vi "Launch Devices to Load Dialog.vi"(8 "error in":errorcluster, 11 "Master Controller in":refnum<class "EMS User Interface.lvclass">) -> (0 "error out":errorcluster, 3 "Master Controller out":refnum<class "EMS User Interface.lvclass">)   [LabVIEW 2018, in "EMS User Interface Actor.lvlib" / "EMS User Interface.lvclass"]
uses:
  EMS User Interface.lvclass
  C:/Users/Administrator/Desktop/LabVIEW EMS/EMS Generic Actor/EMS Generic/EMS Generic.lvclass
  C:/Program Files (x86)/National Instruments/LabVIEW 2018/vi.lib/ActorFramework/Actor/Actor.lvclass
  Dialog Actors/Devices to Load Actor/Devices to Load/Devices to Load.lvclass
  EMS User Interface Messages/Write Device IDs Msg/Write Device IDs Msg.lvclass
  C:/Users/Administrator/Desktop/LabVIEW EMS/Dialog Actors/Devices to Load Actor/Devices to Load Messages/Return Devices to Load IDs Msg/Return Devices to Load IDs Msg.lvclass
  EMS Generic Actor/EMS Generic/EMS Generic.lvclass/EMS Generic.ctl
  EMS User Interface.lvclass/EMS User Interface.ctl
  Dialog Actors/Devices to Load Actor/Devices to Load Messages/Update Device List Msg/Update Device List Msg.lvclass/Update Device List Msg.ctl
  <vilib>/ActorFramework/Message Enqueuer/Message Enqueuer.lvclass/Message Enqueuer.ctl
  <vilib>/ActorFramework/Message Enqueuer/Enqueue.vi
  Dialog Actors/Devices to Load Actor/Devices to Load Messages/Update Device List Msg/Update Device List Msg.lvclass
  C:/Program Files (x86)/National Instruments/LabVIEW 2018/vi.lib/ActorFramework/Message/Message.lvclass
  Global Variables/Global Variables.vi
  <vilib>/ActorFramework/Message Priority Queue/Priority Enqueue.vi
  <vilib>/ActorFramework/Actor/Actor.lvclass
  EMS Generic Actor/EMS Generic/EMS Generic.lvclass
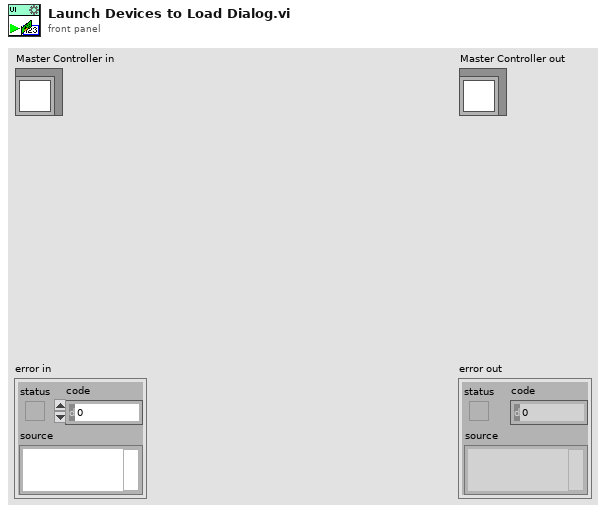
[diagram p1: front panel]
types:
  T1 = typedef "CSEISMIC DDS.lvlib/CSEISMIC DDS.lvclass/DeviceID.ctl" = string
  T2 = typedef "EMS Generic Actor.lvlib/EMS Generic.lvclass/Data Type DVRs.ctl" = cluster{"IED_Status":refnum<data-value>, "IED_Status_0":refnum<data-value>, "DER_Measurement":refnum<data-value>, "DER_Info":refnum<data-value>, "DER_Status":refnum<data-value>, "ES_Measurement":refnum<data-value>, "ES_Info":refnum<data-value>, "PV_Info":refnum<data-value>, "SmartRelay_Info":refnum<data-value>, "SmartRelay_Measurement":refnum<data-value>, "Meter_Info":refnum<data-value>, "Meter_Measurement":refnum<data-value>, "HVAC_Status":refnum<data-value>, "HVAC_Measurement":refnum<data-value>, "PriceData_RealTime":refnum<data-value>, "PriceData_Demand":refnum<data-value>, "PriceData_Energy":refnum<data-value>, "ForecastData_Long":refnum<data-value>, "ForecastData_Short":refnum<data-value>, "DER_Control":refnum<data-value>, "DER_SetPointF":refnum<data-value>, "DER_SetPointP":refnum<data-value>, "DER_SetPointQ":refnum<data-value>, "DER_SetPointPF":refnum<data-value>, "DER_SetPointV":refnum<data-value>, "PV_setCurtailment":refnum<data-value>, "PV_setRampRate":refnum<data-value>, "Relay_Control":refnum<data-value>, "Load_Control":refnum<data-value>, "HVAC_Control":refnum<data-value>, "Generator_Info":refnum<data-value>, "ForecastData_Long_Backup":refnum<data-value>, "PriceData_RealTime_Backup":refnum<data-value>}
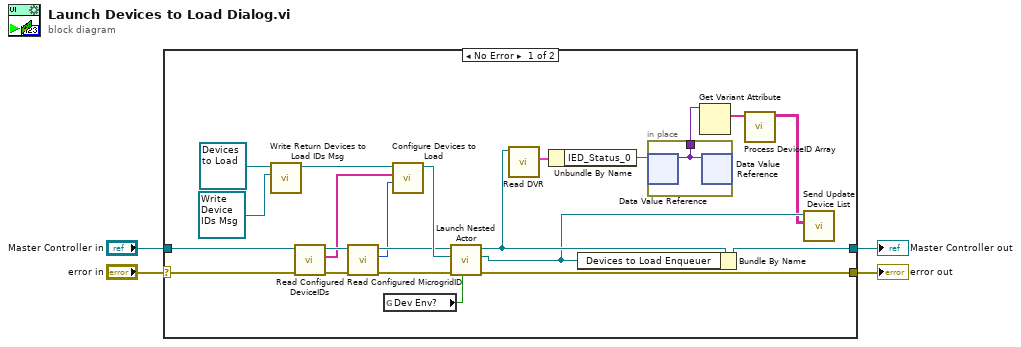
[diagram p0: block diagram]
diagram:
  n1 = case shown="No Error" "error in" {
    selector: "error in" -> [w19 w29]
    tunnel: [w22 w29] -> w3
    tunnel: [w21 w28] -> w1
    tunnel: "Master Controller in" -> [w18 w28]
    frame No Error {
      n2 = call "Write Return Devices to Load IDs Msg.vi"("Return Devices to Load IDs Msg"=refnum<class "Write Device IDs Msg.lvclass"> refnum ("Master Controller Core.lvlib:Write Device IDs Msg.lvclass"), "Devices to Load in"=refnum<class "Devices to Load.lvclass"> refnum ("Devices to Load Config Actor.lvlib:Devices to Load.lvclass")) -> ("Devices to Load out"=w24:refnum<class "Devices to Load.lvclass">)  [unwired: 9 in]
      n3 = call "Read Configured DeviceIDs.vi"("error in"=w19, "EMS Generic in"=w18) -> ("error out"=w14:errorcluster, "DeviceIDs"=w13:T1[], "EMS Generic out"=w17:refnum<class "EMS User Interface.lvclass">)  [unwired: 7 in]
      n4 = call "Read Configured MicrogridID.vi"("error in"=w14, "EMS Generic in"=w17) -> ("error out"=w15:errorcluster, "Microgrid ID"=w12:u8, "EMS Generic out"=w16:refnum<class "EMS User Interface.lvclass">)  [unwired: 7 in]
      n5 = global read "Global Variables.vi" "Dev Env?"() -> (w20:bool)
      n6 = call "Configure Devices to Load.vi"("Microgrid ID"=w12, "Device IDs"=w13, "Devices to Load in"=w24) -> ("Devices to Load out"=w23:refnum<class "Devices to Load.lvclass">)  [unwired: 8 in]
      n7 = call <vilib>:"Launch Nested Actor.vi"("Open Actor Core front panel? (F)"=w20, "error in (no error)"=w15, "Nested Actor"=w23, "Caller Actor in"=w16) -> ("error out"=w22:errorcluster, "Nested Actor's Enqueuer"=w6:refnum<class "Message Enqueuer.lvclass">, "Caller Actor out"=w10:refnum<class "EMS User Interface.lvclass">)  [unwired: 5 in]
      n8 = call "Read DVR.vi"("EMS Generic in"=w10) -> ("DVR"=w11:T2)  [unwired: 9 in, 1 out]
      n9 = Unbundle By Name(w11) -> ("IED_Status_0"=w9:refnum<data-value>)
      n10 = Bundle By Name(cluster=w10, "Devices to Load Enqueuer"=w6) -> (w21:refnum<class "EMS User Interface.lvclass">)
      n11 = in-place {
        in-place-border: [w27] -> w8
        n12 = in-place-dvr #1(w9) -> (w27:variant)  [unwired: 1 out]
        n13 = in-place-dvr #1(w27) -> ()  [unwired: 2 out]
      }
      n14 = Get Variant Attribute(Variant=w8) -> (names=w7:string[])  [unwired: 3 in, 3 out]
      n15 = call "Process DeviceID Array.vi"("DeviceID Array"=w7) -> ("Array"=w5:T1[][])  [unwired: 9 in, 1 out]
      n16 = call "Send Update Device List.vi"("Device Table Strings"=w5, "Message Enqueuer"=w6) -> ()  [unwired: 8 in, 2 out]
    }
    frame Error {
    }
  }
  "error out" <- w3
  "Master Controller out" <- w1
